vi "archive items individually.vi"(1 "suffixes to remove":string[](array[string]), 2 "Array 2":path[](array[path]), 3 "destination folder":path) -> (0 "Errors":errorcluster[](array[cluster]))   [LabVIEW 2009]
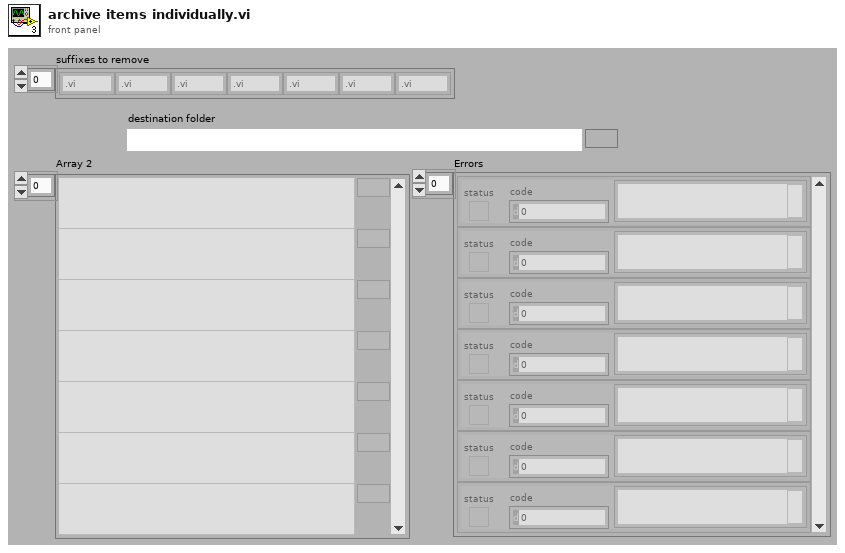
[diagram p1: front panel]
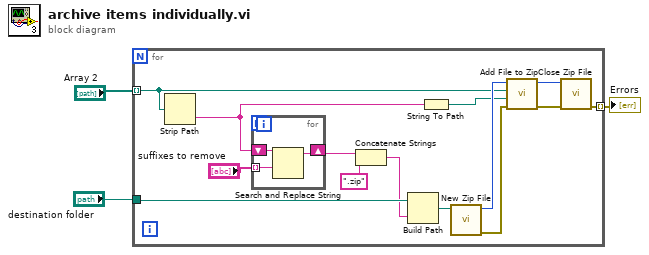
[diagram p0: block diagram]
diagram:
  n1 = for {
    tunnel: "destination folder" -> [w17]
    tunnel: "Array 2" -> [w13] mode=indexing
    tunnel: [w6] -> w2 mode=indexing
    n2 = Strip Path(path=w13) -> (name=w9:string)  [unwired: 1 out]
    n3 = for {
      tunnel: "suffixes to remove" -> [w18] mode=indexing
      shift-right: [w19] -> w5
      shift-left: w9 -> [w20]
      n4 = Search and Replace String(input string=w20, search string=w18) -> (result string=w19:string)  [unwired: 6 in, 3 out]
    }
    n5 = Concatenate Strings(w5, ".zip" ("string")) -> (w11:string)
    n6 = Build Path(base path=w17, name or relative path=w11) -> (appended path=w14:path)
    n7 = String To Path(string=w9) -> (path=w12:path)
    n8 = call <vilib>:"New Zip File.vi"("target"=w14) -> ("error out"=w8:errorcluster, "zip file out"=w16:i64)  [unwired: 4 in, 1 out]
    n9 = call <vilib>:"Add File to Zip.vi"("error in (no error)"=w8, "destination path in zip"=w12, "source file path"=w13, "zip file in"=w16) -> ("error out"=w7:errorcluster, "zip file out"=w15:i64)  [unwired: 6 in]
    n10 = call <vilib>:"Close Zip File.vi"("error in (no error)"=w7, "zip file in"=w15) -> ("error out"=w6:errorcluster)  [unwired: 5 in]
  }
  "Errors" <- w2
